vi "CSPressureSelector.vi"(4 "Scan Period":dbl format="%.2f", 5 "Previous Scan Value":dbl format="%.2f", 6 "Present scan array":dbl[](array[numeric]) format="%.2f", 7 "Value to Output":dbl format="%.2f", 8 "Ch Description":T1={"Ch Name"="", "Type"="", "Function"=enum."Analogue Input", "Ch State"=enum."On", "Calibration type"=enum."Raw", "A"=0.0, "B"=0.0, "C"=0.0, "D"=0.0, "Comments"="", "Address"={"Main"=0, "Ch."=0, "Sub"=0, "Port Name"=""}, "String"="", "Duty"=65535} {"Duty" format="%.0b"; "D" format="%#_5g"; "C" format="%#_5g"; "B" format="%#_5g"; "A" format="%#_5g"}, 9 "Ch names":string[](array[string])) -> (0 "Scan comment":string, 1 "Output":dbl format="%.3f")   [LabVIEW 2014]
doc: "Given an array of Pressure Channels and corresponding Age Channels, this VI evaluates the Age of each Pressure Channel against the Mentos Control Value (minutes). Sufficiently fresh Pressure Channel values are averaged. Stale values are excluded from the average.\n\nThe order of Channels listed in the Comment Field of the Input Channel Description is important: Channels names to average must appear in the comments field separated by semi colons, and each averaging-channel should be immediately preceded by its corresponding Age-Channel. e.g. Comments := \"CSU:Pressure:Age_min;CSU:Pressure:mbar;CFWS:Pressure:Age_min;CFWS:Pressure:mbar\""
uses:
  ADAM_Global.vi
  <vilib>/Analysis/NI_AALBase.lvlib
  <vilib>/Analysis/baseanly.llb/Mean (DBL).vi
  ADAM Client/Sub VIs/ADAM Controls/Function_ADAM.ctl
  ADAM Client/Sub VIs/ADAM Controls/Module_type_ADAM.ctl
  ADAM Client/Sub VIs/ADAM Controls/Address.ctl
  ADAM Client/Sub VIs/ADAM Controls/Ch_description_ADAM.ctl
  ADAM Client/Sub VIs/ADAM Controls/Calib_type_ADAM.ctl
  ADAM Client/Sub VIs/ADAM Controls/Channel_State.ctl
panel:
  in  "Mentos (min)":dbl=60.0
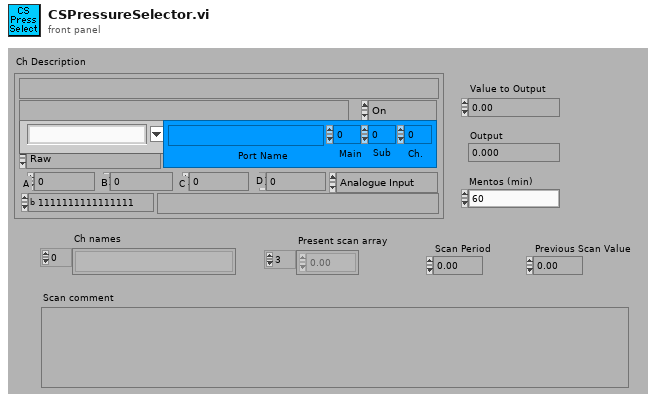
[diagram p1: front panel]
types:
  T1 = typedef "Ch_description_ADAM.ctl" = cluster{"Ch Name":string, "Type":T2, "Function":T3, "Ch State":T4, "Calibration type":T5, "A":dbl, "B":dbl, "C":dbl, "D":dbl, "Comments":string, "Address":T6, "String":string, "Duty":u16}
  T2 = typedef "Module_type_ADAM.ctl" = string
  T3 = typedef "Function_ADAM.ctl" = enum16{"Analogue Input", "Digital Input", "Event counter", "Event rate", "Analogue Output", "Digital Output", "Relay Output"}
  T4 = typedef "Channel_State.ctl" = enum16{"On", "Off", "Always On", "Always Off"}
  T5 = typedef "Calib_type_ADAM.ctl" = enum16{"Raw", "Bx + A", "Cx^2 + Bx + A", "Dx^3 + Cx^2 + Bx + A", "In Band", "Hi-Tec Q", "Hi-Tec M_dot", "Text"}
  T6 = typedef "Address.ctl" = cluster{"Main":i32, "Ch.":i32, "Sub":i32, "Port Name":string}
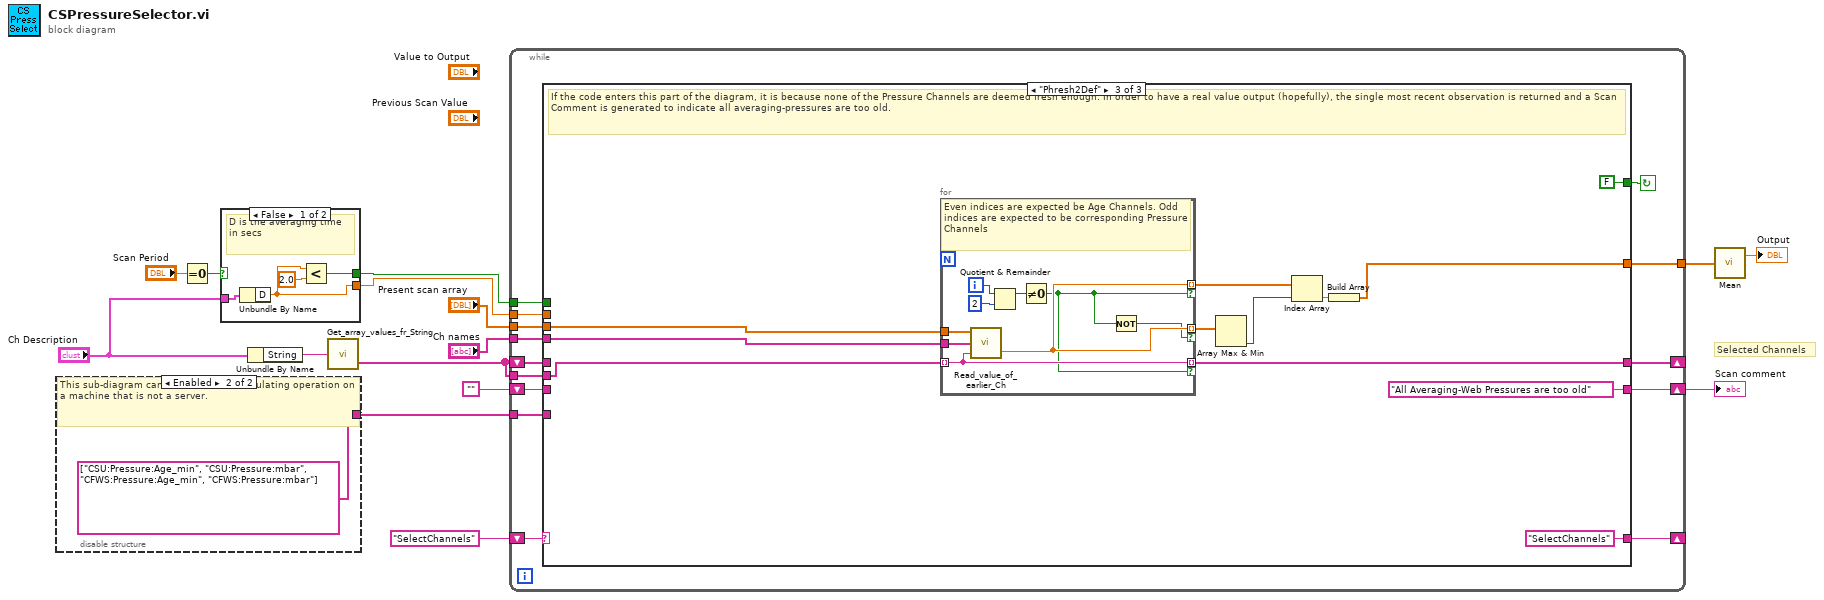
[diagram p0: block diagram]
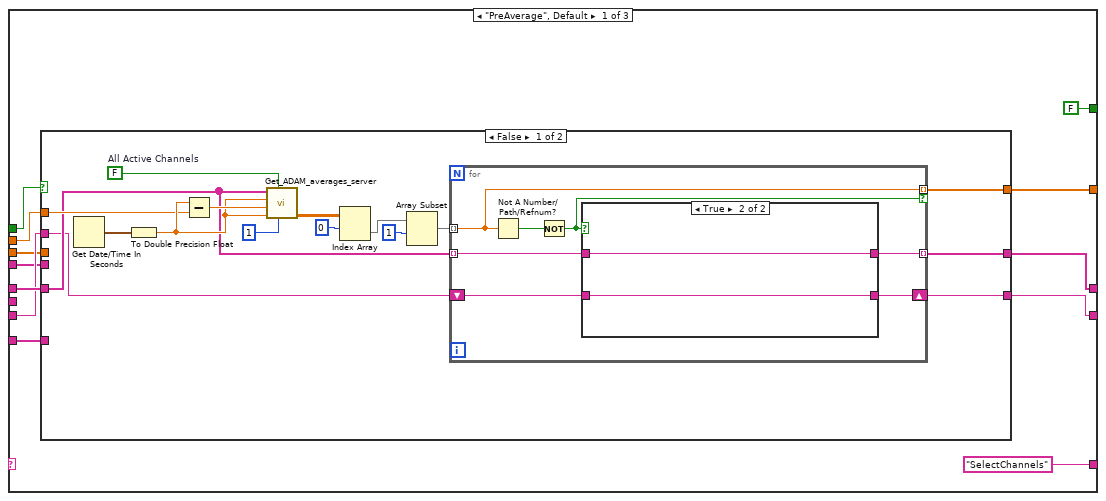
[diagram p2: hidden frame]
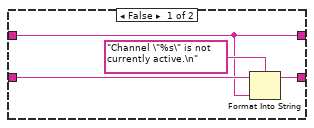
[diagram p3: hidden frame]
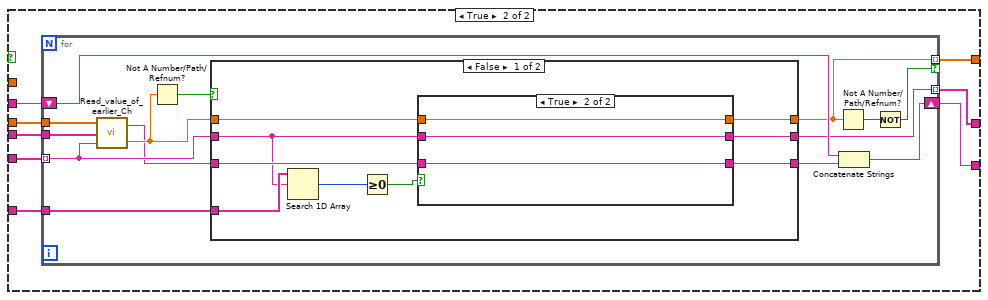
[diagram p4: hidden frame]
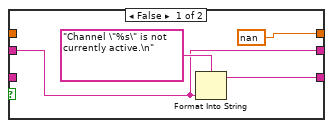
[diagram p5: hidden frame]
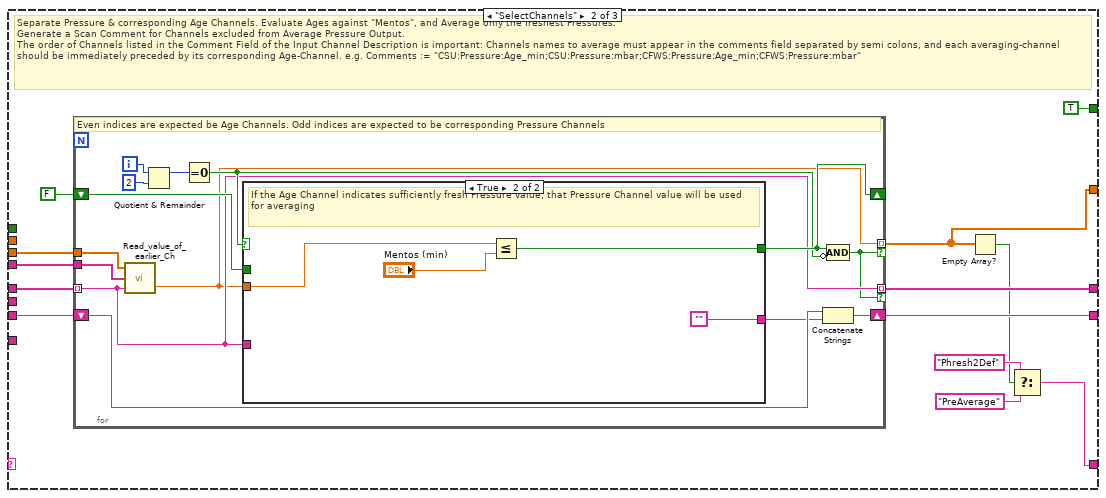
[diagram p7: hidden frame]
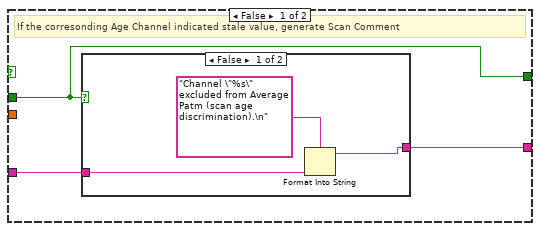
[diagram p8: hidden frame]
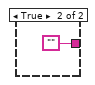
[diagram p9: hidden frame]
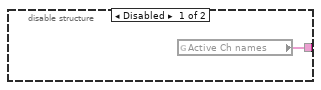
[diagram p10: hidden frame]
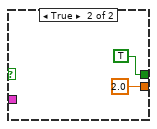
[diagram p11: hidden frame]
diagram:
  # "Selected Channels"
  n1 = disable-structure shown="Enabled" {
    disable-tunnel: [w16 string[] ["CSU:Pressure:Age_min", "CSU:Pressure:mbar", "CFWS:Pressure:Age_min", "CFWS:Pressure:mbar"]] -> w2
    frame Disabled {
      n2 = global read "ADAM_Global.vi" "Active Ch names"() -> (w16:string[])
    }
    frame Enabled {
      # "This sub-diagram can be enabled for simulating operation on a machine that is not a server."
    }
  }
  n3 = Equal To 0?(x="Scan Period") -> (x = 0?=w15:bool)
  n4 = case shown="False" w15 {
    tunnel: "Ch Description" -> [w21 _]
    tunnel: [w19 TRUE] -> w4
    tunnel: [w18 2.0 ("A")] -> w5
    frame False {
      # "D is the averaging time in secs"
      n5 = Unbundle By Name(w21) -> ("D"=w18:dbl)
      n6 = Less?(x=w18, y=2.0) -> (x < y?=w19:bool)
    }
    frame True {
    }
  }
  n7 = Unbundle By Name("Ch Description") -> ("String"=w14:string)
  n8 = call "Get_array_values_fr_String.vi"("String Value"=w14) -> ("String array"=w1:string[])  [unwired: 1 out]
  n9 = while {
    shift-right: [w36] -> _
    shift-left: "SelectChannels" -> [w37]
    tunnel: "Present scan array" -> [w33]
    tunnel: "Ch names" -> [w31]
    shift-right: [w29] -> _
    shift-left: w1 -> [w32]
    tunnel: w5 -> [w28]
    tunnel: w4 -> [w27]
    tunnel: [w26] -> w3
    shift-right: [w30] -> w6
    shift-left: "" -> [w34]
    tunnel: w2 -> [w25]
    tunnel: w1 -> [w24]
    stop <- w35 continue-if-true
    n10 = case shown="\"Phresh2Def\"" w37 {
      tunnel: ["SelectChannels" w122 "SelectChannels"] -> w36
      tunnel: [FALSE TRUE FALSE] -> w35
      tunnel: w34 -> [w42 w131 _]
      tunnel: w33 -> [w39 w130 w167]
      tunnel: w32 -> [w46 w129 _]
      tunnel: w31 -> [w38 w128 w168]
      tunnel: [w47 w125 "All Averaging-Web Pressures are too old"] -> w30
      tunnel: [w41 w126 w165] -> w29
      tunnel: w28 -> [w45 _ _]
      tunnel: w27 -> [w44 _ _]
      tunnel: [w43 w121 w158] -> w26
      tunnel: w25 -> [w40 _ _]
      tunnel: w24 -> [_ _ w163]
      frame "PreAverage", Default {
        n11 = case shown="False" w44 {
          tunnel: w38 -> [_ w86]
          tunnel: w39 -> [_ w85]
          tunnel: w46 -> [w53 w84]
          tunnel: [w52 w83] -> w47
          tunnel: w40 -> [_ w82]
          tunnel: [w54 w81] -> w43
          tunnel: w45 -> [w55 _]
          tunnel: w42 -> [w51 w80]
          tunnel: [w50 w79] -> w41
          frame False {
            w62 = FALSE  # All Active Channels
            n12 = Get Date/Time In Seconds() -> (seconds since 1Jan1904=w65:timestamp)
            n13 = To Double Precision Float(number=w65) -> (double precision float=w63:dbl)
            n14 = Subtract(x=w63, y=w55) -> (x-y=w64:dbl)
            n15 = call "Get_ADAM_averages_server.vi"("No of averages"=1, "All Active Channels"=w62, "End time"=w63, "Start time"=w64, "Clients time"=w63, "ADAM Ch Names"=w53) -> ("DBL values"=w60:dbl[][])  [unwired: 4 out]
            n16 = Index Array(array=w60, index (row)=0) -> (element=w57:dbl[])  [unwired: 1 in]
            n17 = Array Subset(array=w57, index=1) -> (w56:dbl[])  [unwired: 1 in]
            n18 = for {
              tunnel: w56 -> [w72] mode=indexing
              tunnel: [w72] -> w54 mode=indexing if=w70
              tunnel: w53 -> [w69] mode=indexing
              shift-right: [w67] -> w52
              shift-left: w51 -> [w68]
              tunnel: [w66] -> w50 mode=indexing
              n19 = Not A Number/Path/Refnum?(number/path/refnum=w72) -> (NaN/Path/Refnum?=w71:bool)
              n20 = Not(x=w71) -> (.not. x?=w70:bool)
              n21 = case shown="True" w70 {
                tunnel: w69 -> [w73 w77]
                tunnel: w68 -> [w75 w78]
                tunnel: [w74 w78] -> w67
                tunnel: [w73 w77] -> w66
                frame False {
                  n22 = Format Into String(format string="Channel \"%s\" is not currently active.\n", initial string=w75, w73) -> (resulting string=w74:string)  [unwired: 1 in, 1 out]
                }
                frame True {
                }
              }
            }
          }
          frame True {
            n23 = for {
              tunnel: w86 -> [w100]
              tunnel: w85 -> [w99]
              tunnel: w84 -> [w96] mode=indexing
              shift-right: [w97] -> w83
              shift-left: w80 -> [w98]
              tunnel: [w90] -> w81 mode=indexing if=w88
              tunnel: w82 -> [w91]
              tunnel: [w87] -> w79 mode=indexing
              n24 = call "Read_value_of_earlier_Ch.vi"("Desired Ch to Read"=w96, "Ch names"=w100, "Present scan array"=w99) -> ("Value"=w94:dbl, "Scan comment"=w93:string)  [unwired: 1 in]
              n25 = Not A Number/Path/Refnum?(number/path/refnum=w94) -> (NaN/Path/Refnum?=w95:bool)
              n26 = case shown="False" w95 {
                tunnel: w96 -> [w104 w117]
                tunnel: [w107 w119] -> w90
                tunnel: w94 -> [w106 w119]
                tunnel: [w109 w118] -> w92
                tunnel: w93 -> [w108 w118]
                tunnel: w91 -> [w105 _]
                tunnel: [w101 w117] -> w87
                frame False {
                  n27 = Search 1D Array(1D array=w105, element=w104) -> (index of element=w102:i32)  [unwired: 1 in]
                  n28 = Greater Or Equal To 0?(x=w102) -> (x >= 0?=w103:bool)
                  n29 = case shown="True" w103 {
                    tunnel: w104 -> [w110 w114]
                    tunnel: [w113 w116] -> w109
                    tunnel: w108 -> [_ w116]
                    tunnel: [nan w115] -> w107
                    tunnel: w106 -> [_ w115]
                    tunnel: [w110 w114] -> w101
                    frame False {
                      n30 = Format Into String(format string="Channel \"%s\" is not currently active.\n", w110) -> (resulting string=w113:string)  [unwired: 2 in, 1 out]
                    }
                    frame True {
                    }
                  }
                }
                frame True {
                }
              }
              n31 = Not A Number/Path/Refnum?(number/path/refnum=w90) -> (NaN/Path/Refnum?=w89:bool)
              n32 = Concatenate Strings(w98, w92) -> (w97:string)
              n33 = Not(x=w89) -> (.not. x?=w88:bool)
            }
          }
        }
      }
      frame "SelectChannels" {
        # "Separate Pressure & corresponding Age Channels. Evaluate Ages against \"Mentos\", and Average only the freshest Pressures.\nGenerate a Scan Comment for Channels excluded from Average Pressure Output.\nThe order of Channels listed in the Comment Field of the Input Channel Description is important: Channels names to average must appear in the comments field separated by semi colons, and each averaging-channel should be immediately preceded by its corresponding Age-Channel. e.g. Comments := \"CSU:Pressure:Age_min;CSU:Pressure:mbar;CFWS:Pressure:Age_min;CFWS:Pressure:mbar\""
        n34 = for {
          shift-right: [w142] -> _
          shift-left: FALSE -> [w143]
          tunnel: [w137] -> w126 mode=indexing if=w133
          tunnel: w130 -> [w140]
          tunnel: w129 -> [w137] mode=indexing
          shift-right: [w139] -> w125
          shift-left: w131 -> [w138]
          tunnel: w128 -> [w135]
          tunnel: [w134] -> w121 mode=indexing if=w133
          i -> [w146]
          # "Even indices are expected be Age Channels. Odd indices are expected to be corresponding Pressure Channels"
          n35 = call "Read_value_of_earlier_Ch.vi"("Desired Ch to Read"=w137, "Ch names"=w135, "Present scan array"=w140) -> ("Value"=w134:dbl)  [unwired: 1 in, 1 out]
          n36 = Quotient & Remainder(x=w146, y=2) -> (x-y*floor(x/y)=w144:i32)  [unwired: 1 out]
          n37 = Equal To 0?(x=w144) -> (x = 0?=w141:bool)
          n38 = case shown="True" w141 {
            tunnel: [w149 w156] -> w142
            tunnel: w143 -> [w149 _]
            tunnel: w134 -> [_ w155]
            tunnel: w137 -> [w148 _]
            tunnel: [w147 ""] -> w136
            frame False {
              # "If the corresonding Age Channel indicated stale value, generate Scan Comment"
              n39 = case shown="False" w149 {
                tunnel: w148 -> [w151 _]
                tunnel: [w150 ""] -> w147
                frame False {
                  n40 = Format Into String(format string="Channel \"%s\" excluded from Average Patm (scan age discrimination).\n", w151) -> (resulting string=w150:string)  [unwired: 2 in, 1 out]
                }
                frame True {
                }
              }
            }
            frame True {
              # "If the Age Channel indicates sufficiently fresh Pressure value, that Pressure Channel value will be used for averaging"
              n41 = Less Or Equal?(x=w155, y="Mentos (min)") -> (x <= y?=w156:bool)
            }
          }
          n42 = Concatenate Strings(w138, w136) -> (w139:string)
          n43 = Compound Arithmetic op=AND(w142, invert w141) -> (w133:bool)
        }
        n44 = Empty Array?(array=w121) -> (empty?=w120:bool)
        n45 = Select(t="Phresh2Def", s=w120, f="PreAverage") -> (s? t:f=w122:string)
      }
      frame "Phresh2Def" {
        # "If the code enters this part of the diagram, it is because none of the Pressure Channels are deemed fresh enough. In order to have a real value output (hopefully), the single most recent observation is returned and a Scan Comment is generated to indicate all averaging-pressures are too old."
        n46 = for {
          tunnel: [w174] -> w165 mode=indexing if=w171
          tunnel: w167 -> [w175]
          tunnel: w163 -> [w174] mode=indexing
          tunnel: w168 -> [w173]
          tunnel: [w172] -> w161 mode=indexing if=w171
          tunnel: [w172] -> w162 mode=indexing if=w170
          i -> [w178]
          # "Even indices are expected be Age Channels. Odd indices are expected to be corresponding Pressure Channels"
          n47 = call "Read_value_of_earlier_Ch.vi"("Desired Ch to Read"=w174, "Ch names"=w173, "Present scan array"=w175) -> ("Value"=w172:dbl)  [unwired: 1 in, 1 out]
          n48 = Quotient & Remainder(x=w178, y=2) -> (x-y*floor(x/y)=w176:i32)  [unwired: 1 out]
          n49 = Not Equal To 0?(x=w176) -> (x != 0?=w171:bool)
          n50 = Not(x=w171) -> (.not. x?=w170:bool)
        }
        n51 = Array Max & Min(array=w162) -> (min index (indices)=w160:i32)  [unwired: 3 out]
        n52 = Index Array(array=w161, index=w160) -> (element=w159:dbl)
        n53 = Build Array(w159) -> (w158:dbl[])
      }
    }
  }
  "Scan comment" <- w6
  n54 = call-poly <vilib>:"Mean.vi"("X"=w3) -> ("mean"=→"Output":dbl)  [unwired: 1 out]
